vi "Selected Row Axis Read.vi"(4 "error in (no error)":errorcluster, 6 "Container State":T4, 7 "Display State In":T1={"Initialization"=TRUE, "Show in and out values"=TRUE, "Show Highliting"=TRUE, "Open Plot"=FALSE, "Format String"="%10_4g", "X"=0.0, "Y"=0.0, "Limits"={"Min X"=inf, "Max X"=inf, "MaxDiff X"=inf, "MaxGrad X"=inf, "Min Y"=inf, "Max Y"=inf, "MaxDiff Y"=inf, "MaxGrad Y"=inf, "Min Z"=inf, "Max Z"=inf, "MaxDiff Z"=inf}, "Vertical Scrollbar"=FALSE, "Horizontal Scrollbar"=FALSE, "Data"={"X"=[1.0, 2.0], "Y"=[3.0, 4.0], "Z"=[[5.0, 7.0], [6.0, 8.0]]}, "Undo Avaliable"=FALSE, "NIVS System Definition Root"=refnum, "Selected Parameter 2D"="", "Selected Working Pt 2D"=[], "Z"=0.0, "Row Axis"="", "Col Axis"=""}) -> (0 "error out":errorcluster, 2 "Value":string, 3 "Display State Out":T1={"Initialization"=TRUE, "Show in and out values"=TRUE, "Show Highliting"=TRUE, "Open Plot"=FALSE, "Format String"="%10_4g", "X"=0.0, "Y"=0.0, "Limits"={"Min X"=inf, "Max X"=inf, "MaxDiff X"=inf, "MaxGrad X"=inf, "Min Y"=inf, "Max Y"=inf, "MaxDiff Y"=inf, "MaxGrad Y"=inf, "Min Z"=inf, "Max Z"=inf, "MaxDiff Z"=inf}, "Vertical Scrollbar"=FALSE, "Horizontal Scrollbar"=FALSE, "Data"={"X"=[1.0, 2.0], "Y"=[3.0, 4.0], "Z"=[[5.0, 7.0], [6.0, 8.0]]}, "Undo Avaliable"=FALSE, "NIVS System Definition Root"=refnum, "Selected Parameter 2D"="", "Selected Working Pt 2D"=[], "Z"=0.0, "Row Axis"="", "Col Axis"=""})   [LabVIEW 2011, in "TBL2D.xctl"]
uses:
  TBL2D.xctl
  <vilib>/_xctls/Container State.ctl
  State TBL2D.ctl
  Limits TBL2D.ctl
  Data TBL2D.ctl
  NationalInstruments.VeriStand.SystemStorage
  <vilib>/_xctls/XControlSupport.lvlib
panel:
  # "Replace the Value Indicator below with an Indicator of desired type.\nDo not remove this Indicator or the others from the connector pane. \nDo not change the connector pane pattern.\nThe Value Indicator should always be the second terminal from top on the output side in the connector pane."
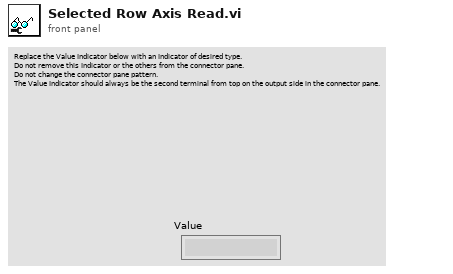
[diagram p1: front panel]
types:
  T1 = typedef "TBL2D.xctl/State TBL2D.ctl" = cluster{"Initialization":bool, "Show in and out values":bool, "Show Highliting":bool, "Open Plot":bool, "Format String":string, "X":sgl, "Y":sgl, "Limits":T2, "Vertical Scrollbar":bool, "Horizontal Scrollbar":bool, "Data":T3, "Undo Avaliable":bool, "NIVS System Definition Root":refnum<k24>, "Selected Parameter 2D":string, "Selected Working Pt 2D":string[], "Z":sgl, "Row Axis":string, "Col Axis":string}
  T2 = typedef "TBL2D.xctl/Limits TBL2D.ctl" = cluster{"Min X":sgl, "Max X":sgl, "MaxDiff X":sgl, "MaxGrad X":sgl, "Min Y":sgl, "Max Y":sgl, "MaxDiff Y":sgl, "MaxGrad Y":sgl, "Min Z":sgl, "Max Z":sgl, "MaxDiff Z":sgl}
  T3 = typedef "TBL2D.xctl/Data TBL2D.ctl" = cluster{"X":sgl[], "Y":sgl[], "Z":sgl[][]}
  T4 = typedef "XControlSupport.lvlib/Container State.ctl" = cluster{"Indicator?":bool, "Run Mode?":bool, " Refnum":refnum<vi>}
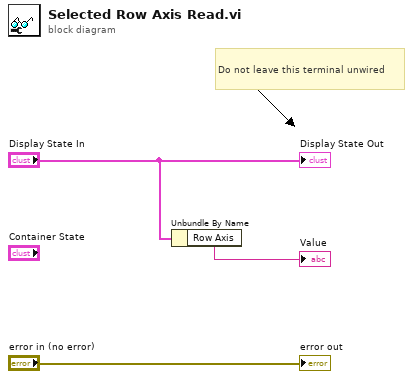
[diagram p0: block diagram]
diagram:
  # "Do not leave this terminal unwired"
  n1 = Unbundle By Name("Display State In") -> ("Row Axis"=→"Value":string)
  "error out" <- "error in (no error)"
  "Display State Out" <- "Display State In"
